vi "Property Tree Set Value_Master.vi"(7 "Action":T1, 8 "Error In":errorcluster, 9 "Tag Selected":string[](array[string]), 10 "Active Tree":refnum<vi>, 11 "All Tree Refs":refnum<vi>[](array[refnum])) -> (0 "Error Out":errorcluster)   [LabVIEW 2023]
doc: "Toggle has already happened, so here we determine if row is selecgted and deal with updating the tree value"
uses:
  controls/action enum.ctl
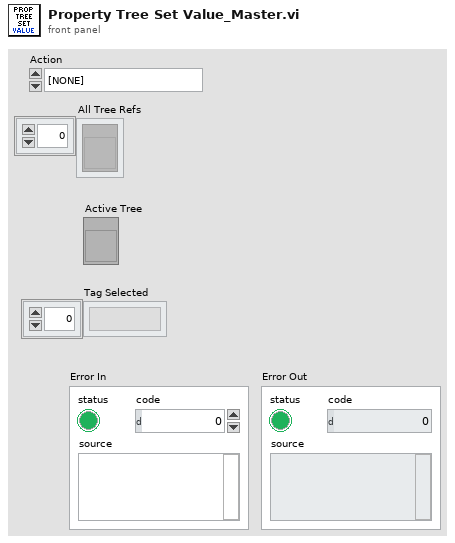
[diagram p1: front panel]
types:
  T1 = typedef "action enum.ctl" = enum16{"[NONE]", "Wire Bundle", "Wire Unbundle", "Terminal Unbundle", "Terminal Bundle", "Bundler Move Up", "Bundler Move Down", "Bundler Insert", "Bundler Remove", "Bundler Remove Unwired", "Bundler Rearrange", "In Place Insert", "In Place Remove", "In Place Remove Unwired", "In Place Rearrange", "Wire Properties", "Wire Method", "Terminal Properties", "Terminal Method", "Property Move Up", "Property Move Down", "Properties Insert", "Properties Remove", "Properties Remove Unwired", "Properties Rearrange", "Method Change", "Class for Constant", "Class For Control", "Class For Node", "Class Name to Clipboard"}
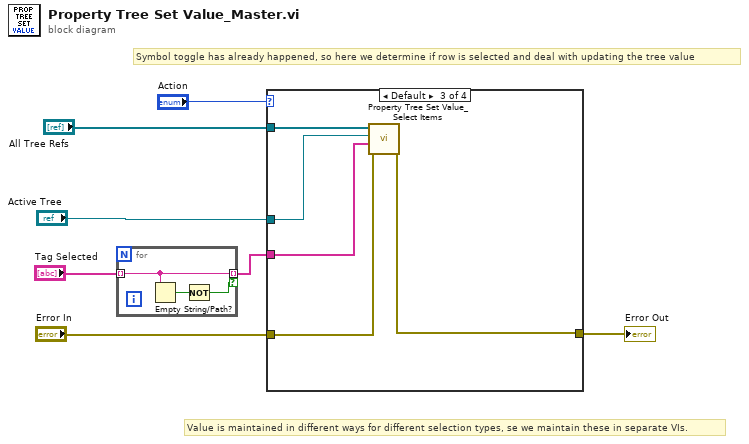
[diagram p0: block diagram]
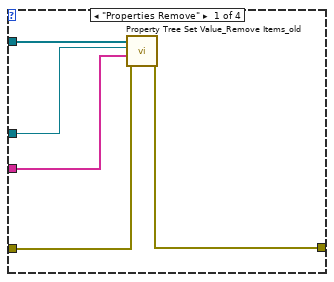
[diagram p2: hidden frame]
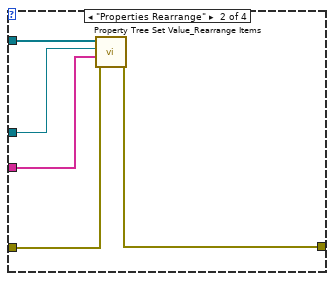
[diagram p3: hidden frame]
diagram:
  # "Value is maintained in different ways for different selection types, se we maintain these in separate VIs."
  # "Symbol toggle has already happened, so here we determine if row is selected and deal with updating the tree value"
  n1 = for {
    tunnel: "Tag Selected" -> [w10] mode=indexing
    tunnel: [w10] -> w1 mode=indexing if=w8
    n2 = Empty String/Path?(string/path=w10) -> (empty?=w9:bool)
    n3 = Not(x=w9) -> (.not. x?=w8:bool)
  }
  n4 = case shown="Default" "Action" {
    tunnel: "Active Tree" -> [w13 w18 w23 _]
    tunnel: w1 -> [w14 w19 w24 _]
    tunnel: "All Tree Refs" -> [w15 w20 w25 _]
    tunnel: "Error In" -> [w12 w16 w22 w26]
    tunnel: [w11 w17 w21 w26] -> w3
    frame "Properties Remove" {
      n5 = call "Property Tree Set Value_Remove Items_old.vi"("Error In"=w12, "Tag Selected"=w14, "Active Tree"=w13, "All Tree Refs"=w15) -> ("Error Out"=w11:errorcluster)  [unwired: 7 in]
    }
    frame "Properties Rearrange" {
      n6 = call "Property Tree Set Value_Rearrange Items.vi"("Error In"=w16, "Tag Selected"=w19, "Active Tree"=w18, "All Tree Refs"=w20) -> ("Error Out"=w17:errorcluster)  [unwired: 7 in]
    }
    frame Default {
      n7 = call "Property Tree Set Value_Select Items.vi"("Error In"=w22, "Tag Selected"=w24, "Active Tree"=w23, "All Tree Refs"=w25) -> ("Error Out"=w21:errorcluster)  [unwired: 7 in]
    }
    frame "Wire Method", "Terminal Method", "Method Change" {
      # "use tree iteself for value"
    }
  }
  "Error Out" <- w3
